vi "Test Lockin Digitizer.vi"(8 "error in":errorcluster) -> ()   [LabVIEW 2021]
uses:
  Instruments/Pulse Driver/Lockin Digitizer Driver/Lockin Digitizer Configuration.ctl
  <vilib>/DAQmx/write.llb/DAQmx Write (Analog 1D DBL 1Chan NSamp).vi
  <vilib>/DAQmx/read.llb/DAQmx Read (Analog 2D DBL NChan NSamp).vi
  <vilib>/Analysis/2dsp.llb/Decimate (single shot, DBL).vi
  <vilib>/DAQmx/create/channels.llb/DAQmx Create Channel (AO-Voltage-Basic).vi
  <vilib>/DAQmx/create/channels.llb/DAQmx Create Channel (AI-Voltage-Basic).vi
  <vilib>/DAQmx/configure/timing.llb/DAQmx Timing (Sample Clock).vi
  <vilib>/DAQmx/configure/trigger.llb/DAQmx Start Trigger (None).vi
  <vilib>/DAQmx/configure/trigger.llb/DAQmx Reference Trigger (Digital Edge).vi
  <vilib>/DAQmx/miscellaneous.llb/DAQmx Fill In Error Info.vi
  <resource>/objmgr/daqmx.rc
  <vilib>/Analysis/NI_AALBase.lvlib
  <vilib>/Analysis/NI_AALPro.lvlib
panel:
  in  "Configuration":T1={"Post-trigger delay"=0.01, "Post-trigger duration"=0.1, "Rate"=1000000.0, "Ranges"=[10.0], "Re-name channels"=[], "Active channels"="0:1", "External\nclock"=FALSE, "Frequencies"=[100000.0], "Time\nconstant"=1.0, "Output \namplitudes"=[1.0], "Input\nchannles"=["0"]} {"Output \namplitudes" format="%#_6pV"; "Time\nconstant" format="%#_6ps"; "Frequencies" format="%#_6pHz"; "Rate" format="%#_8pHz"; "Post-trigger duration" format="%#_6ps"; "Post-trigger delay" format="%#_6ps"; "Ranges" format="%#_6pV"}
  out "data":dbl[][](array[numeric])
  out "size(s)":i32[](array[numeric])
  in  "Plot raw":bool
  out "Output buffer":u32
  in  "Output pre-buffers #":i32=4
  out "AvailSampPerChan":u32
  in  "DAQmx Device Name":tag
  in  "Lock-in":bool
  in  "buffer size (in samples per channel)":u32=1000000 format="%.0p"
  in  "Phase shift":dbl
  out "Waveform Chart":dbl[][](graph)
  in  "decimating factor":i32=1
  out "x = 0?":bool
  in  "number of samples per channel":i32=100000 format="%.6p"
  out "Cycle":i32
  in  "timeout":dbl=1.0 format="%0.2f"
  in  "AI samples per channel":i32=1000
  out "Waveform Graph":cluster{dbl, dbl, "data":dbl[][]}(graph)
  out "Actual sample rate":dbl format="%#_6p"
  in  "pretrigger samples per channel":u32=500
  out "Done":bool
  in  "Stop Button":bool
  # "Digitizer config"
  # "Lock-in config"
  # "#0\n\n#1"
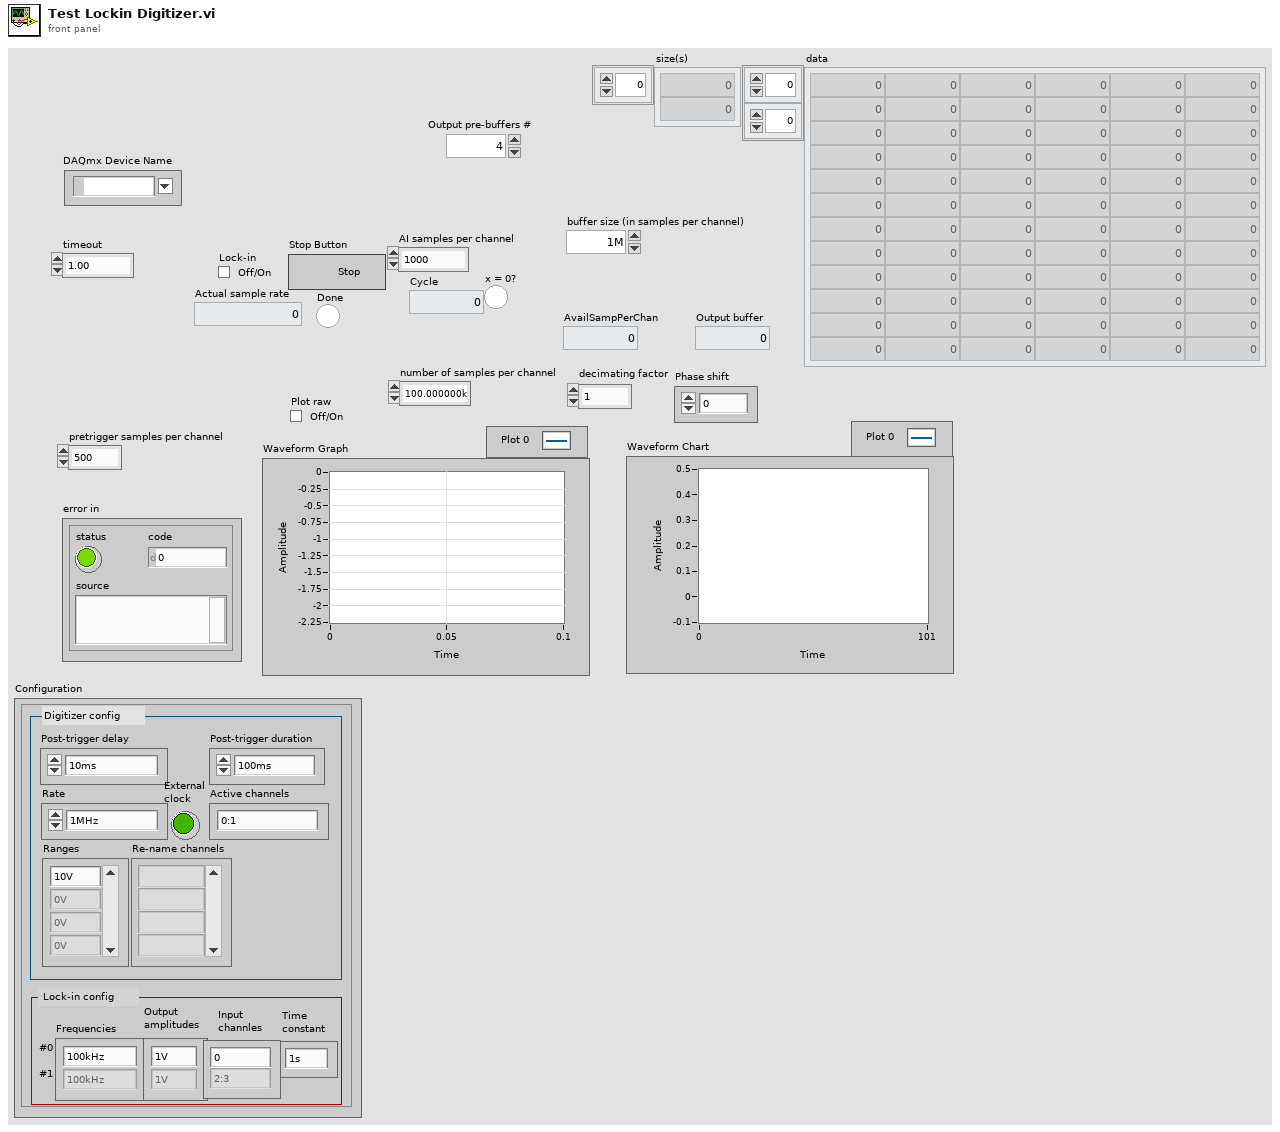
[diagram p1: front panel]
types:
  T1 = typedef "Lockin Digitizer Configuration.ctl" = cluster{"Post-trigger delay":dbl, "Post-trigger duration":dbl, "Rate":dbl, "Ranges":dbl[], "Re-name channels":string[], "Active channels":string, "External\nclock":bool, "Frequencies":dbl[], "Time\nconstant":dbl, "Output \namplitudes":dbl[], "Input\nchannles":string[]}
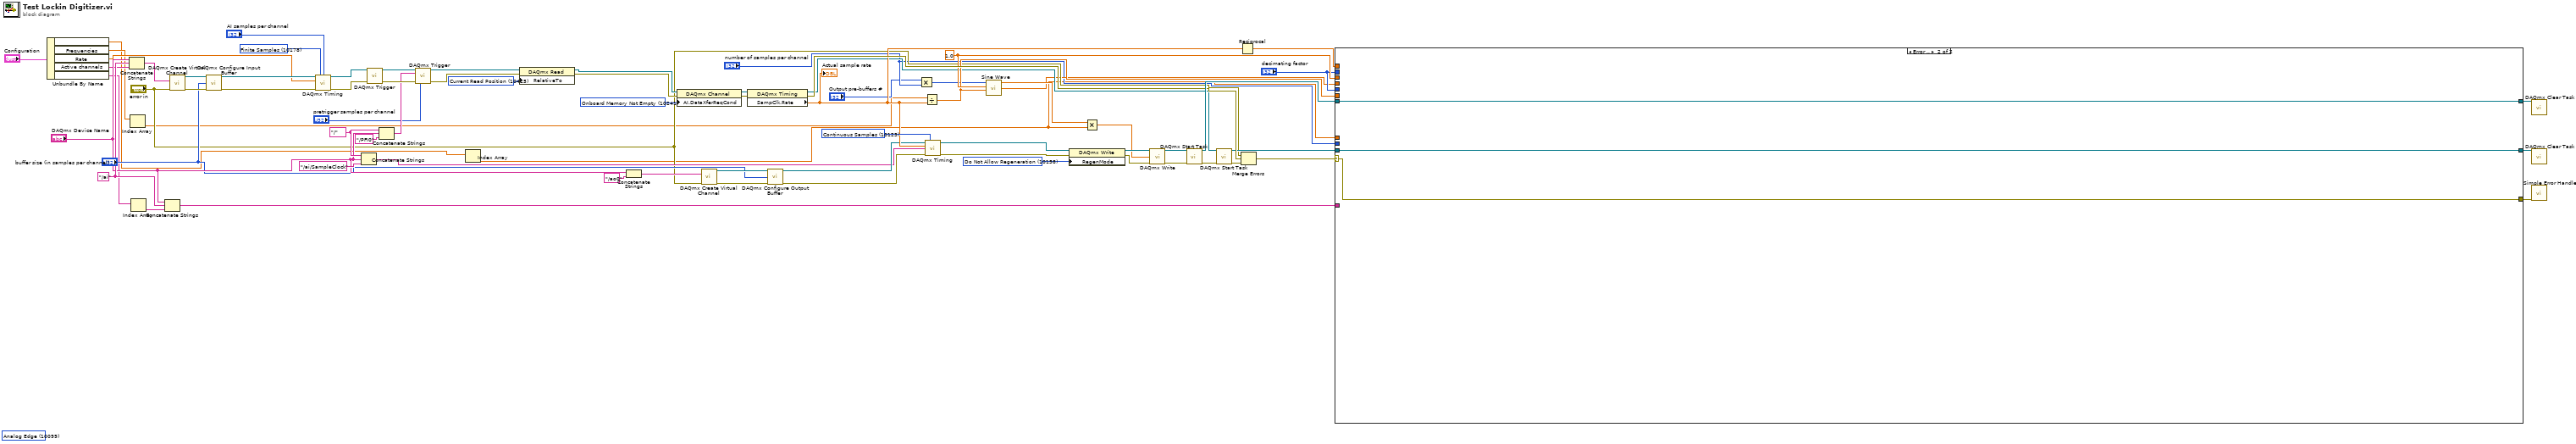
[diagram p0: block diagram]
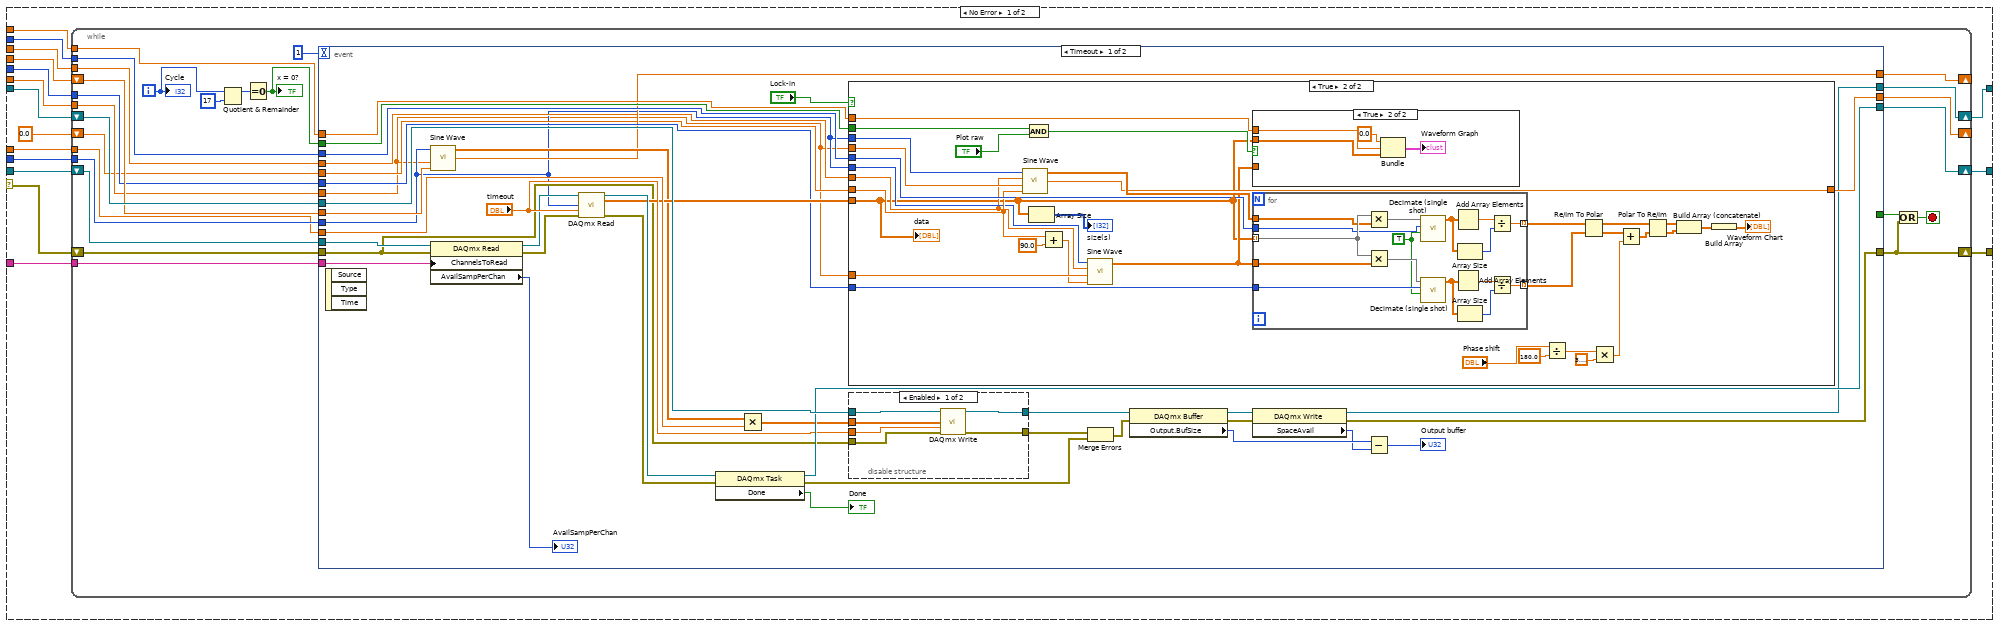
[diagram p2: hidden frame]
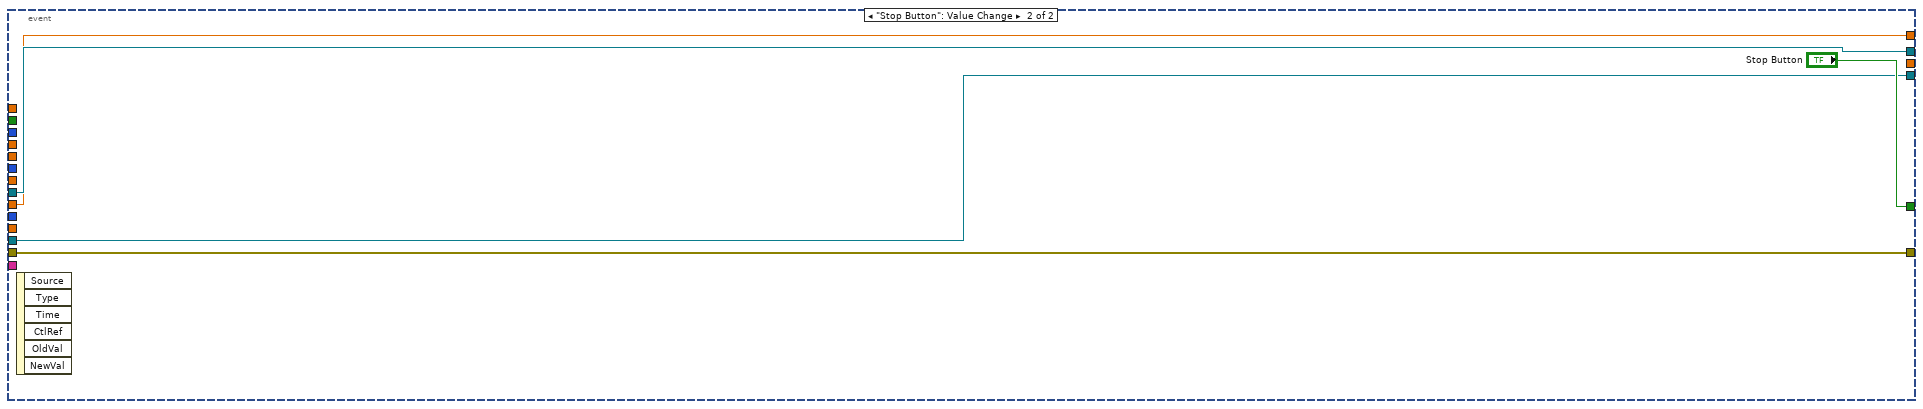
[diagram p6: hidden frame]
diagram:
  w21 = tag "/" ("string")
  w20 = "/ai" ("string")
  w42 = 1.0
  w52 = 10425 items=["First Sample"=10424, "Current Read Position"=10425, "Reference Trigger"=10426, "First Pretrigger Sample"=10427, "Most Recent Sample"=10428] ("RelativeTo")
  w59 = 10241 items=["Onboard Memory More than Half Full"=10237, "Onboard Memory Not Empty"=10241, "Onboard Memory Custom Threshold"=12577, "When Acquisition Complete"=12546] ("AI.DataXferReqCond")
  w65 = 10123 items=["Finite Samples"=10178, "Continuous Samples"=10123, "Hardware Timed Single Point"=12522] ("sample mode")
  w66 = 10178 items=["Finite Samples"=10178, "Continuous Samples"=10123, "Hardware Timed Single Point"=12522] ("sample mode")
  w72 = 10158 items=["Allow Regeneration"=10097, "Do Not Allow Regeneration"=10158] ("RegenMode")
  (unwired) 10099 items=["Analog Edge"=10099, "Analog Multi Edge"=16108, "Digital Edge"=10150, "Digital Pattern"=10398, "Analog Window"=10103, "Time"=15996, "None"=10230] ("Start.TrigType")
  n1 = Unbundle By Name("Configuration") -> ("Output \namplitudes"=w2:dbl[], "Frequencies"=w4:dbl[], "Rate"=w8:dbl, "Active channels"=w6:string, "Input\nchannles"=w7:string[])
  n2 = Concatenate Strings("DAQmx Device Name", w20, w6) -> (w26:string)
  n3 = Index Array(array=w4) -> (element=w3:dbl)  [unwired: 1 in]
  n4 = Index Array(array=w7) -> (element=w5:string)  [unwired: 1 in]
  n5 = Concatenate Strings("DAQmx Device Name", w20, w5) -> (w14:string)
  n6 = call-poly <vilib>:"DAQmx Create Virtual Channel.vi"("physical channels"=w26, "error in"="error in") -> ("task out"=w48:refnum<k21>, "error out"=w47:errorcluster)  [unwired: 12 in]
  n7 = call <vilib>:"DAQmx Configure Input Buffer.vi"("task/channels in"=w48, "buffer size (in samples per channel)"="buffer size (in samples per channel)", "error in"=w47) -> ("task out"=w46:refnum<k21>, "error out"=w45:errorcluster)  [unwired: 11 in]
  n8 = call-poly <vilib>:"DAQmx Timing.vi"("task/channels in"=w46, "sample mode"=w66, "samples per channel"="AI samples per channel", "rate"=w8, "error in"=w45) -> ("task out"=w57:refnum<k21>, "error out"=w55:errorcluster)  [unwired: 9 in]
  n9 = Concatenate Strings(w21, "DAQmx Device Name", "/ai/SampleClock" ("string")) -> (w22:string)
  n10 = call-poly <vilib>:"DAQmx Trigger.vi"("task/channels in"=w57, "error in"=w55) -> ("task out"=w56:refnum<k21>, "error out"=w54:errorcluster)  [unwired: 12 in]
  n11 = Concatenate Strings(w21, "DAQmx Device Name", "/PFI0" ("string")) -> (w16:string)
  n12 = call-poly <vilib>:"DAQmx Trigger.vi"("task/channels in"=w56, "source"=w16, "error in"=w54, "pretrigger samples per channel"="pretrigger samples per channel") -> ("task out"=w53:refnum<k21>, "error out"=w51:errorcluster)  [unwired: 10 in]
  n13 = Index Array(array=w2) -> (element=w1:dbl)  [unwired: 1 in]
  n14 = property class="DAQmx Read"(reference=w53, error in=w51, "RelativeTo"=w52) -> (reference out=w50:refnum<k21>, error out=w49:errorcluster)
  n15 = Concatenate Strings("DAQmx Device Name", "/ao0" ("string")) -> (w24:string)
  n16 = property class="DAQmx Channel"(reference=w50, error in=w49, "AI.DataXferReqCond"=w59) -> (reference out=w37:refnum<k21>, error out=w36:errorcluster)
  n17 = call-poly <vilib>:"DAQmx Create Virtual Channel.vi"("physical channels"=w24, "error in"="error in") -> ("task out"=w31:refnum<k21>, "error out"=w30:errorcluster)  [unwired: 12 in]
  n18 = property class="DAQmx Timing"(reference=w37, error in=w36) -> (reference out=w33:refnum<k21>, error out=w58:errorcluster, "SampClk.Rate"=w44:dbl)
  "Actual sample rate" <- w44
  n19 = call <vilib>:"DAQmx Configure Output Buffer.vi"("task/channels in"=w31, "buffer size (in samples per channel)"="buffer size (in samples per channel)", "error in"=w30) -> ("task out"=w28:refnum<k21>, "error out"=w29:errorcluster)  [unwired: 11 in]
  n20 = Multiply(x="Output pre-buffers #", y="number of samples per channel") -> (x*y=w11:i32)
  n21 = Divide(x=w3, y=w44) -> (x/y=w41:dbl)
  n22 = call-poly <vilib>:"DAQmx Timing.vi"("task/channels in"=w28, "sample mode"=w65, "rate"=w44, "source"=w22, "error in"=w29) -> ("task out"=w73:refnum<k21>, "error out"=w74:errorcluster)  [unwired: 9 in]
  n23 = call <vilib>:"Sine Wave.vi"("samples"=w11, "amplitude"=w42, "frequency"=w41) -> ("sine wave"=w39:dbl[], "phase out"=w13:dbl)  [unwired: 2 in, 1 out]
  n24 = property class="DAQmx Write"(reference=w73, error in=w74, "RegenMode"=w72) -> (reference out=w68:refnum<k21>, error out=w67:errorcluster)
  n25 = Multiply(x=w39, y=w1) -> (x*y=w38:dbl[])
  n26 = call-poly <vilib>:"DAQmx Write.vi"("task/channels in"=w68, "data"=w38, "error in"=w67) -> ("task out"=w69:refnum<k21>, "error out"=w70:errorcluster)  [unwired: 10 in, 1 out]
  n27 = call <vilib>:"DAQmx Start Task.vi"("task/channels in"=w69, "error in"=w70) -> ("task out"=w71:refnum<k21>, "error out"=w35:errorcluster)  [unwired: 12 in]
  n28 = call <vilib>:"DAQmx Start Task.vi"("task/channels in"=w33, "error in"=w35) -> ("task out"=w32:refnum<k21>, "error out"=w34:errorcluster)  [unwired: 12 in]
  n29 = Reciprocal(x=w44) -> (1/x=w43:dbl)
  n30 = Merge Errors("error in", w58, w34) -> (w60:errorcluster)
  n31 = case shown="Error .." w60 {
    selector: w60 -> [w87 w224]
    tunnel: [w90 w224] -> w61
    tunnel: w71 -> [w89 w223]
    tunnel: w32 -> [w88 w222]
    tunnel: [w86 w223] -> w63
    tunnel: [w85 w222] -> w62
    tunnel: "number of samples per channel" -> [w84 _]
    tunnel: w13 -> [w83 _]
    tunnel: w43 -> [w82 _]
    tunnel: w41 -> [w81 _]
    tunnel: w42 -> [w80 _]
    tunnel: w1 -> [w79 _]
    tunnel: "decimating factor" -> [w78 _]
    tunnel: "decimating factor" -> [w77 _]
    tunnel: w14 -> [w76 _]
    frame No Error {
      n32 = while {
        shift-right: [w111] -> w90
        shift-left: w87 -> [w113]
        shift-right: [w109] -> w86
        shift-left: w89 -> [w110]
        shift-right: [w107] -> w85
        shift-left: w88 -> [w108]
        tunnel: w84 -> [w106]
        shift-right: [w103] -> _
        shift-left: w83 -> [w104]
        tunnel: w82 -> [w105]
        tunnel: w81 -> [w99]
        tunnel: w80 -> [w98]
        tunnel: w79 -> [w96]
        tunnel: w78 -> [w95]
        tunnel: w77 -> [w94]
        tunnel: w76 -> [w93]
        shift-right: [w91] -> _
        shift-left: 0.0 ("phase in") -> [w92]
        i -> [w102]
        stop <- w112 stop-if-true
        n33 = Quotient & Remainder(x=w102, y=17) -> (x-y*floor(x/y)=w97:i32)  [unwired: 1 out]
        n34 = Equal To 0?(x=w97) -> (x = 0?=w100:bool)
        "x = 0?" <- w100
        n35 = event shown="[0] Timeout" {
          selector: _ -> [_ _]
          dyn-events: _ -> [_ _]
          timeout: 1 -> [_ _]
          tunnel: [_ "Stop Button"] -> w115
          tunnel: w113 -> [w134 w219]
          tunnel: [w123 w219] -> w111
          tunnel: w110 -> [w153 w220]
          tunnel: [w124 w220] -> w109
          tunnel: w108 -> [w137 w218]
          tunnel: [w150 w218] -> w107
          tunnel: w106 -> [w126 _]
          tunnel: w105 -> [w147 _]
          tunnel: w104 -> [w131 w217]
          tunnel: [w130 w217] -> w103
          tunnel: w100 -> [w146 _]
          tunnel: w99 -> [w125 _]
          tunnel: w98 -> [w129 _]
          tunnel: w96 -> [w145 _]
          tunnel: w95 -> [w142 _]
          tunnel: w94 -> [w141 _]
          tunnel: w93 -> [w136 _]
          tunnel: w92 -> [w128 _]
          tunnel: [w127 _] -> w91
          event Timeout {
            n36 = event-data() -> ()  [unwired: 1 in, 3 out]
            n37 = call <vilib>:"Sine Wave.vi"("samples"=w126, "frequency"=w125, "phase in"=w131) -> ("sine wave"=w132:dbl[], "phase out"=w130:dbl)  [unwired: 2 in, 1 out]
            n38 = property class="DAQmx Read"(reference=w137, error in=w134, "ChannelsToRead"=w136) -> (reference out=w138:refnum<k21>, error out=w135:errorcluster, "AvailSampPerChan"=→"AvailSampPerChan":u32)
            n39 = call-poly <vilib>:"DAQmx Read.vi"("task/channels in"=w138, "number of samples per channel"=w126, "timeout"="timeout", "error in"=w135) -> ("task out"=w151:refnum<k21>, "data"=w143:dbl[][], "error out"=w148:errorcluster)  [unwired: 9 in]
            n40 = property class="DAQmx Task"(reference=w151, error in=w148) -> (reference out=w150:refnum<k21>, error out=w154:errorcluster, "Done"=→"Done":bool)
            n41 = Multiply(x=w132, y=w145) -> (x*y=w144:dbl[])
            n42 = case shown="True" "Lock-in" {
              tunnel: w147 -> [_ w188]
              tunnel: w146 -> [_ w158]
              tunnel: w143 -> [_ w157]
              tunnel: w142 -> [_ w187]
              tunnel: w141 -> [_ w186]
              tunnel: w126 -> [_ w173]
              tunnel: w129 -> [_ w167]
              tunnel: w125 -> [_ w172]
              tunnel: w128 -> [w155 w169]
              tunnel: [w155 w170] -> w127
              tunnel: w126 -> [_ w168]
              tunnel: w125 -> [_ w166]
              frame False {
              }
              frame True {
                n43 = call <vilib>:"Sine Wave.vi"("samples"=w173, "amplitude"=w167, "frequency"=w172, "phase in"=w169) -> ("sine wave"=w171:dbl[], "phase out"=w170:dbl)  [unwired: 1 in, 1 out]
                n44 = And(x=w158, y="Plot raw") -> (x .and. y?=w159:bool)
                n45 = Array Size(array=w157) -> (size(s)=→"size(s)":i32[])
                n46 = Add(x=w169, y=90.0 ("phase in")) -> (x+y=w163:dbl)
                n47 = call <vilib>:"Sine Wave.vi"("samples"=w168, "amplitude"=w167, "frequency"=w166, "phase in"=w163) -> ("sine wave"=w165:dbl[])  [unwired: 1 in, 2 out]
                n48 = case shown="True" w159 {
                  tunnel: w188 -> [_ w190]
                  tunnel: w157 -> [_ w192]
                  tunnel: w165 -> [_ _]
                  frame False {
                  }
                  frame True {
                    n49 = Bundle(0.0, w190, "data"=w192) -> (→"Waveform Graph":cluster{dbl, dbl, "data":dbl[][]})  [unwired: 1 in]
                  }
                }
                n50 = for {
                  tunnel: w157 -> [w208] mode=indexing
                  tunnel: w171 -> [w207]
                  tunnel: w187 -> [w205]
                  tunnel: w186 -> [w202]
                  tunnel: [w195] -> w161 mode=indexing
                  tunnel: [w194] -> w162 mode=indexing
                  tunnel: w165 -> [w193]
                  w203 = TRUE ("averaging")
                  n51 = Multiply(x=w208, y=w207) -> (x*y=w204:dbl[])
                  n52 = Multiply(x=w208, y=w193) -> (x*y=w206:dbl[])
                  n53 = call-poly <vilib>:"Decimate (single shot).vi"("averaging"=w203, "decimating factor"=w202, "X"=w204) -> ("Decimated Array"=w196:dbl[])  [unwired: 7 in, 1 out]
                  n54 = call-poly <vilib>:"Decimate (single shot).vi"("averaging"=w203, "decimating factor"=w205, "X"=w206) -> ("Decimated Array"=w201:dbl[])  [unwired: 7 in, 1 out]
                  n55 = Add Array Elements(numeric array=w196) -> (sum=w198:dbl)
                  n56 = Add Array Elements(numeric array=w201) -> (sum=w199:dbl)
                  n57 = Array Size(array=w196) -> (size(s)=w197:i32)
                  n58 = Array Size(array=w201) -> (size(s)=w200:i32)
                  n59 = Divide(x=w198, y=w197) -> (x/y=w194:dbl)
                  n60 = Divide(x=w199, y=w200) -> (x/y=w195:dbl)
                }
                n61 = Divide(x="Phase shift", y=180.0) -> (x/y=w180:dbl)
                n62 = Re/Im To Polar(2:w161, 3:w162) -> (0:w183:dbl[], 1:w178:dbl[])
                n63 = Multiply(x=w180, y=3.141592653589793) -> (x*y=w177:dbl)
                n64 = Add(x=w183, y=w177) -> (x+y=w176:dbl[])
                n65 = Polar To Re/Im(2:w176, 3:w178) -> (0:w174:dbl[], 1:w175:dbl[])
                n66 = Build Array (concatenate)(w175, w174) -> (w185:dbl[])
                n67 = Build Array(w185) -> (→"Waveform Chart":dbl[][])
                "data" <- w157
              }
            }
            n68 = disable-structure shown="Enabled" {
              disable-tunnel: w153 -> [w214 w215]
              disable-tunnel: [w213 w216] -> w152
              disable-tunnel: [w212 w215] -> w122
              disable-tunnel: w144 -> [w211 _]
              disable-tunnel: "timeout" -> [w210 _]
              disable-tunnel: w134 -> [w209 w216]
              frame Enabled {
                n69 = call-poly <vilib>:"DAQmx Write.vi"("task/channels in"=w214, "data"=w211, "timeout"=w210, "error in"=w209) -> ("task out"=w212:refnum<k21>, "error out"=w213:errorcluster)  [unwired: 9 in, 1 out]
              }
              frame Disabled {
              }
            }
            n70 = Merge Errors(w152, w154) -> (w117:errorcluster)
            n71 = property class="DAQmx Buffer"(reference=w122, error in=w117) -> (reference out=w118:refnum<k21>, error out=w116:errorcluster, "Output.BufSize"=w121:u32)
            n72 = property class="DAQmx Write"(reference=w118, error in=w116) -> (reference out=w124:refnum<k21>, error out=w123:errorcluster, "SpaceAvail"=w120:u32)
            n73 = Subtract(x=w121, y=w120) -> (x-y=→"Output buffer":u32)
          }
          event "Stop Button": Value Change {
            n74 = event-data() -> ()  [unwired: 1 in, 6 out]
          }
        }
        n75 = Or(x=w115, y=w111) -> (x .or. y?=w112:bool)
        "Cycle" <- w102
      }
    }
    frame Error {
    }
  }
  n76 = call <vilib>:"DAQmx Clear Task.vi"("task in"=w63) -> ()  [unwired: 14 in, 1 out]
  n77 = call <vilib>:"DAQmx Clear Task.vi"("task in"=w62) -> ()  [unwired: 14 in, 1 out]
  n78 = call <vilib>:"Simple Error Handler.vi"("error in (no error)"=w61) -> ()  [unwired: 4 in, 5 out]
